vi "AutoProgramState.vi"(3 "error in (no error)":errorcluster, 4 "INcluster":T1, 6 "G-Code Array":string[](array[string])) -> (0 "error in (no error) 2":errorcluster, 1 "Stop State":bool, 2 "Next Command":string)   [LabVIEW 2017]
uses:
  libraryGcode/control/Queue/QueueCMDandPOS.ctl
  libraryGcode/control/UartCmdQueueUpdate.ctl
  libraryGcode/control/StateMachineAuto.ctl
  libraryGcode/ClassStateAuto/StateAuto.lvclass
  controls/state_board_control.ctl
  global/GLOBAL_STATE.vi
  libraryGcode/LibraryGcode.lvlib
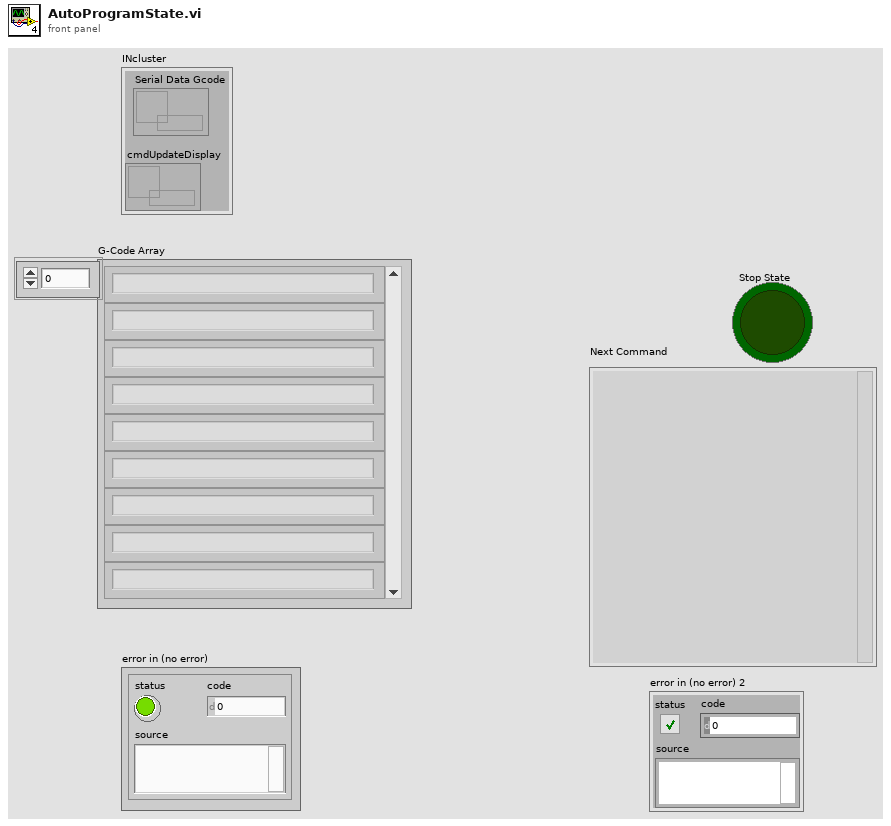
[diagram p1: front panel]
types:
  T1 = typedef "QueueCMDandPOS.ctl" = cluster{"Serial Data Gcode":refnum<queue>, "cmdUpdateDisplay":refnum<queue>}
  T2 = typedef "LibraryGcode.lvlib/StateMachineAuto.ctl" = enum16{"init", "checkEMG", "checkStateBoard", "checkQueue", "writeDataQueue", "initNextCommand", "endNextCommand"}
  T3 = typedef "state_board_control.ctl" = enum16{"Running", "Waiting", "Pos", "IDLE"}
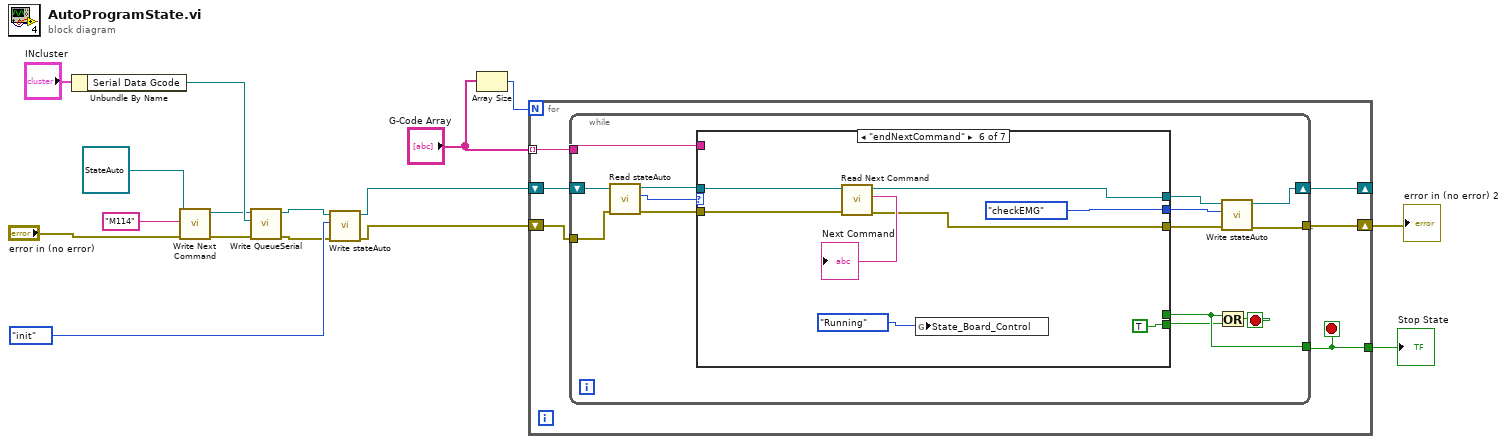
[diagram p0: block diagram]
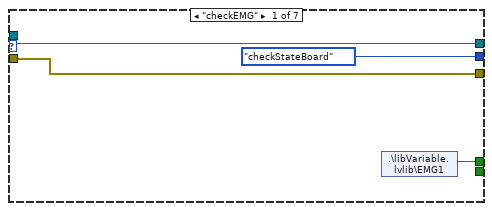
[diagram p2: hidden frame]
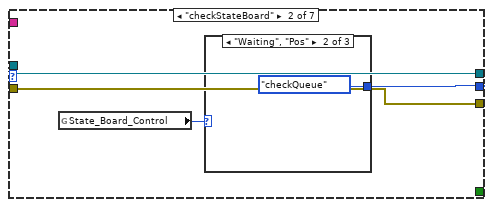
[diagram p3: hidden frame]
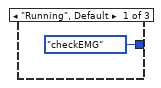
[diagram p4: hidden frame]
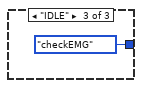
[diagram p5: hidden frame]
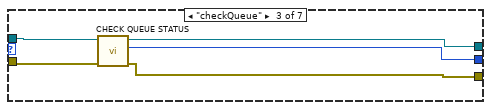
[diagram p6: hidden frame]
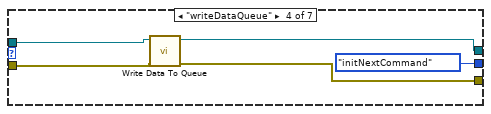
[diagram p7: hidden frame]
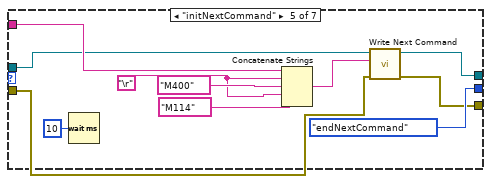
[diagram p8: hidden frame]
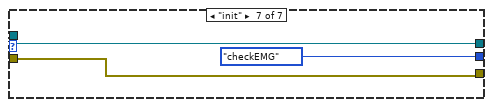
[diagram p9: hidden frame]
diagram:
  n1 = Unbundle By Name("INcluster") -> ("Serial Data Gcode"=w11:refnum<queue>)
  n2 = call-dynamic "Write Next Command.vi"("error in (no error)"="error in (no error)", "Next Command"="M114", "StateAuto in"=refnum<class "StateAuto.lvclass"> refnum) -> ("error out"=w5:errorcluster, "StateAuto out"=w9:refnum<class "StateAuto.lvclass">)  [unwired: 7 in]
  n3 = call-dynamic "Write QueueSerial.vi"("error in (no error)"=w5, "QueueSerial"=w11, "StateAuto in"=w9) -> ("error out"=w4:errorcluster, "StateAuto out"=w8:refnum<class "StateAuto.lvclass">)  [unwired: 7 in]
  n4 = call-dynamic "Write stateAuto.vi"("error in (no error)"=w4, "Enum"=StateMachineAuto."init", "StateAuto in"=w8) -> ("error out"=w3:errorcluster, "StateAuto out"=w7:refnum<class "StateAuto.lvclass">)  [unwired: 7 in]
  n5 = Array Size(array="G-Code Array") -> (size(s)=w15:i32)
  n6 = for {
    N: w15 -> [_]
    tunnel: "G-Code Array" -> [w22] mode=indexing
    tunnel: [w21] -> w13
    shift-right: [w19] -> _
    shift-left: w7 -> [w20]
    shift-right: [w17] -> w1
    shift-left: w3 -> [w18]
    stop <- w21 stop-if-true
    n7 = while {
      tunnel: w22 -> [w36]
      tunnel: [w35] -> w21
      shift-right: [w23] -> w19
      shift-left: w20 -> [w32]
      tunnel: w18 -> [w28]
      tunnel: [w27] -> w17
      stop <- w34 stop-if-true
      n8 = call-dynamic "Read stateAuto.vi"("error in (no error)"=w28, "StateAuto in"=w32) -> ("error out"=w24:errorcluster, "Enum"=w30:T2, "StateAuto out"=w31:refnum<class "StateAuto.lvclass">)  [unwired: 7 in]
      n9 = case shown="\"endNextCommand\"" w30 {
        tunnel: w36 -> [_ _ _ _ w66 _ _]
        tunnel: [w38 _ _ _ _ _ _] -> w35
        tunnel: [_ _ _ _ _ TRUE ("y") _] -> w33
        tunnel: [w37 w41 w50 w53 w60 w70 w77] -> w26
        tunnel: w31 -> [w40 w43 w52 w56 w61 w74 w79]
        tunnel: [w40 w43 w49 w54 w59 w69 w79] -> w29
        tunnel: [StateMachineAuto."checkStateBoard" ("Enum") w42 w48 StateMachineAuto."initNextCommand" ("Enum") StateMachineAuto."endNextCommand" ("Enum") StateMachineAuto."checkEMG" ("Enum") StateMachineAuto."checkEMG" ("Enum")] -> w25
        tunnel: w24 -> [w37 w41 w51 w55 w58 w71 w77]
        frame "checkEMG" {
          n10 = shared-variable ".\\libVariable.lvlib\\EMG1"() -> (w38:bool)  [unwired: 1 in, 1 out]
        }
        frame "checkStateBoard" {
          n11 = global read "GLOBAL_STATE.vi" "State_Board_Control"() -> (w44:T3)
          n12 = case shown="\"Waiting\", \"Pos\"" w44 {
            tunnel: [StateMachineAuto."checkEMG" ("Enum") StateMachineAuto."checkQueue" ("Enum") StateMachineAuto."checkEMG" ("Enum")] -> w42
            frame "Running", Default {
            }
            frame "Waiting", "Pos" {
            }
            frame "IDLE" {
            }
          }
        }
        frame "checkQueue" {
          n13 = call-dynamic "CHECK QUEUE STATUS.vi"("error in (no error)"=w51, "StateAuto in"=w52) -> ("error out"=w50:errorcluster, "stateAuto"=w48:T2, "StateAuto out"=w49:refnum<class "StateAuto.lvclass">)  [unwired: 7 in]
        }
        frame "writeDataQueue" {
          n14 = call-dynamic "Write Data To Queue.vi"("error in (no error)"=w55, "StateAuto in"=w56) -> ("error out"=w53:errorcluster, "StateAuto out"=w54:refnum<class "StateAuto.lvclass">)  [unwired: 8 in]
        }
        frame "initNextCommand" {
          w65 = "\r"
          n15 = Wait (ms)(milliseconds to wait=u32 10) -> ()  [unwired: 1 out]
          n16 = Concatenate Strings(w66, w65, "M400" ("string"), w65, "M114" ("string")) -> (w63:string)
          n17 = call-dynamic "Write Next Command.vi"("error in (no error)"=w58, "Next Command"=w63, "StateAuto in"=w61) -> ("error out"=w60:errorcluster, "StateAuto out"=w59:refnum<class "StateAuto.lvclass">)  [unwired: 7 in]
        }
        frame "endNextCommand" {
          n18 = call-dynamic "Read Next Command.vi"("error in (no error)"=w71, "StateAuto in"=w74) -> ("error out"=w70:errorcluster, "Next Command"=→"Next Command":string, "StateAuto out"=w69:refnum<class "StateAuto.lvclass">)  [unwired: 7 in]
          n19 = global write "GLOBAL_STATE.vi" "State_Board_Control"(state_board_control."Running" ("state_board_STM1")) -> ()
        }
        frame "init" {
        }
      }
      n20 = Or(x=w35, y=w33) -> (x .or. y?=w34:bool)
      n21 = call-dynamic "Write stateAuto.vi"("error in (no error)"=w26, "Enum"=w25, "StateAuto in"=w29) -> ("error out"=w27:errorcluster, "StateAuto out"=w23:refnum<class "StateAuto.lvclass">)  [unwired: 7 in]
    }
  }
  "Stop State" <- w13
  "error in (no error) 2" <- w1
